vi "Google Earth.vi"() -> ()   [LabVIEW 2014]
uses:
  <vilib>/Instr/_visa.llb/VISA Configure Serial Port (Instr).vi
panel:
  out "Light":dbl(slide) scale=0.0..3000.0
  in  "Body Movements":T1
  out "Audio":dbl(slide) scale=0.0..30000.0
  out "x = y?":bool
  in  "Stop Button":bool
  in  "Globe Params":T2={"Longitude"=0.0, "Latitude"=0.0, "Altitude"=15000000.0, "Azimuth"=0.0}
  in  "Globe":refnum<k7>(container)
  in  "EARTHLib.IApplicationGE 2":refnum<k7>
  # "Space Glove Interface"
  # "Earth View"
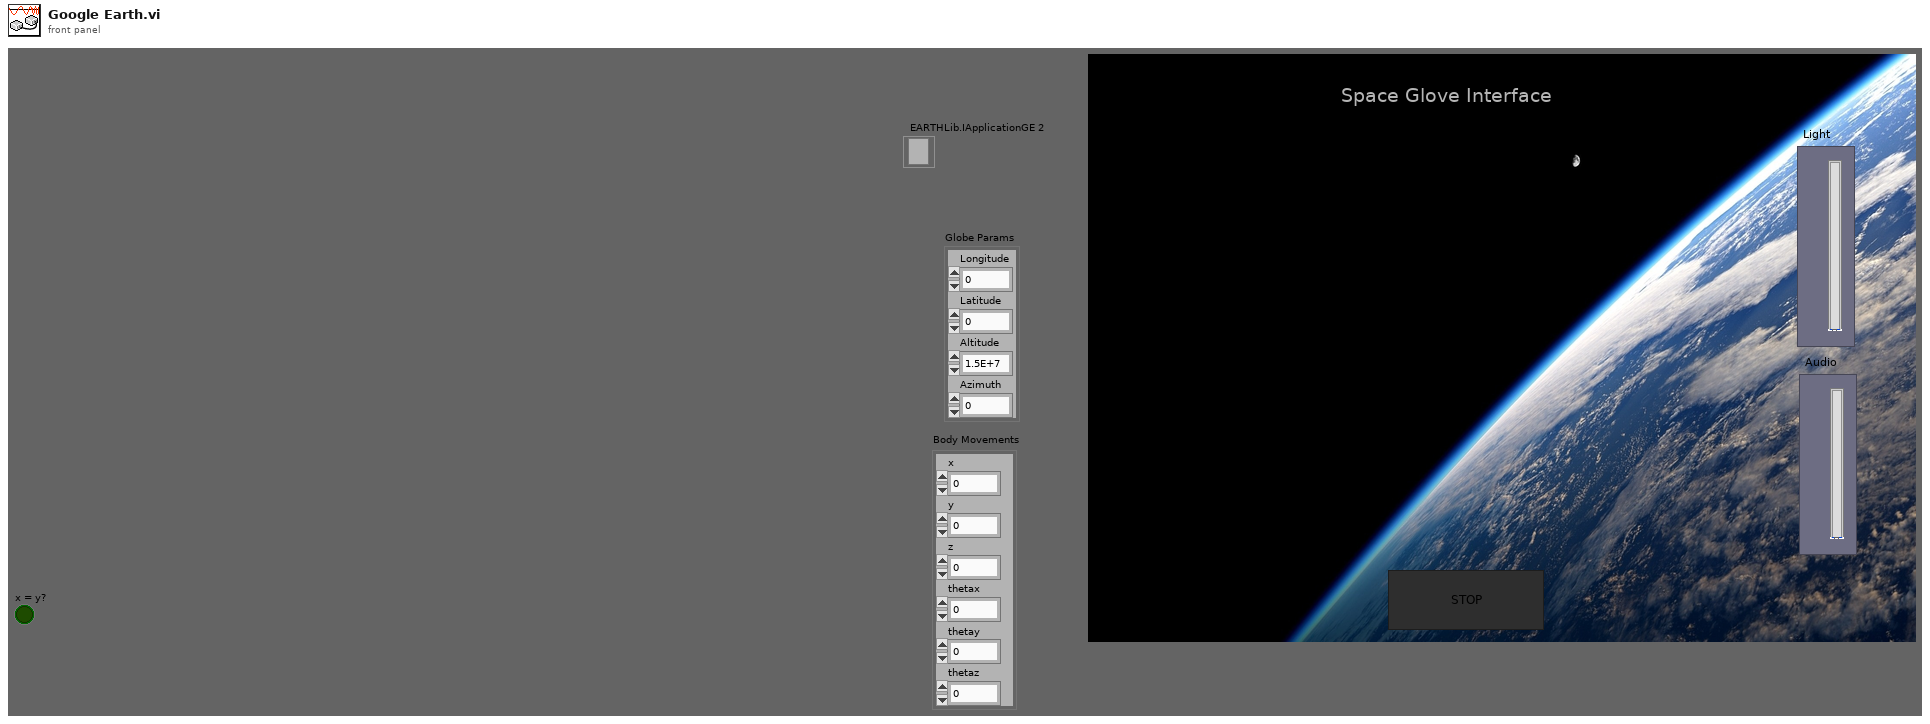
[diagram p1: front panel]
types:
  T1 = cluster{"x":sgl, "y":sgl, "z":sgl, "thetax":sgl, "thetay":sgl, "thetaz":sgl}
  T2 = cluster{"Longitude":dbl, "Latitude":dbl, "Altitude":dbl, "Azimuth":dbl}
  T3 = cluster{"Azimuth":dbl, "FocusPointAltitude":dbl, "altMode":i32, "FocusPointLatitude":dbl, "FocusPointLongitude":dbl, "Range":dbl, "Tilt":dbl}
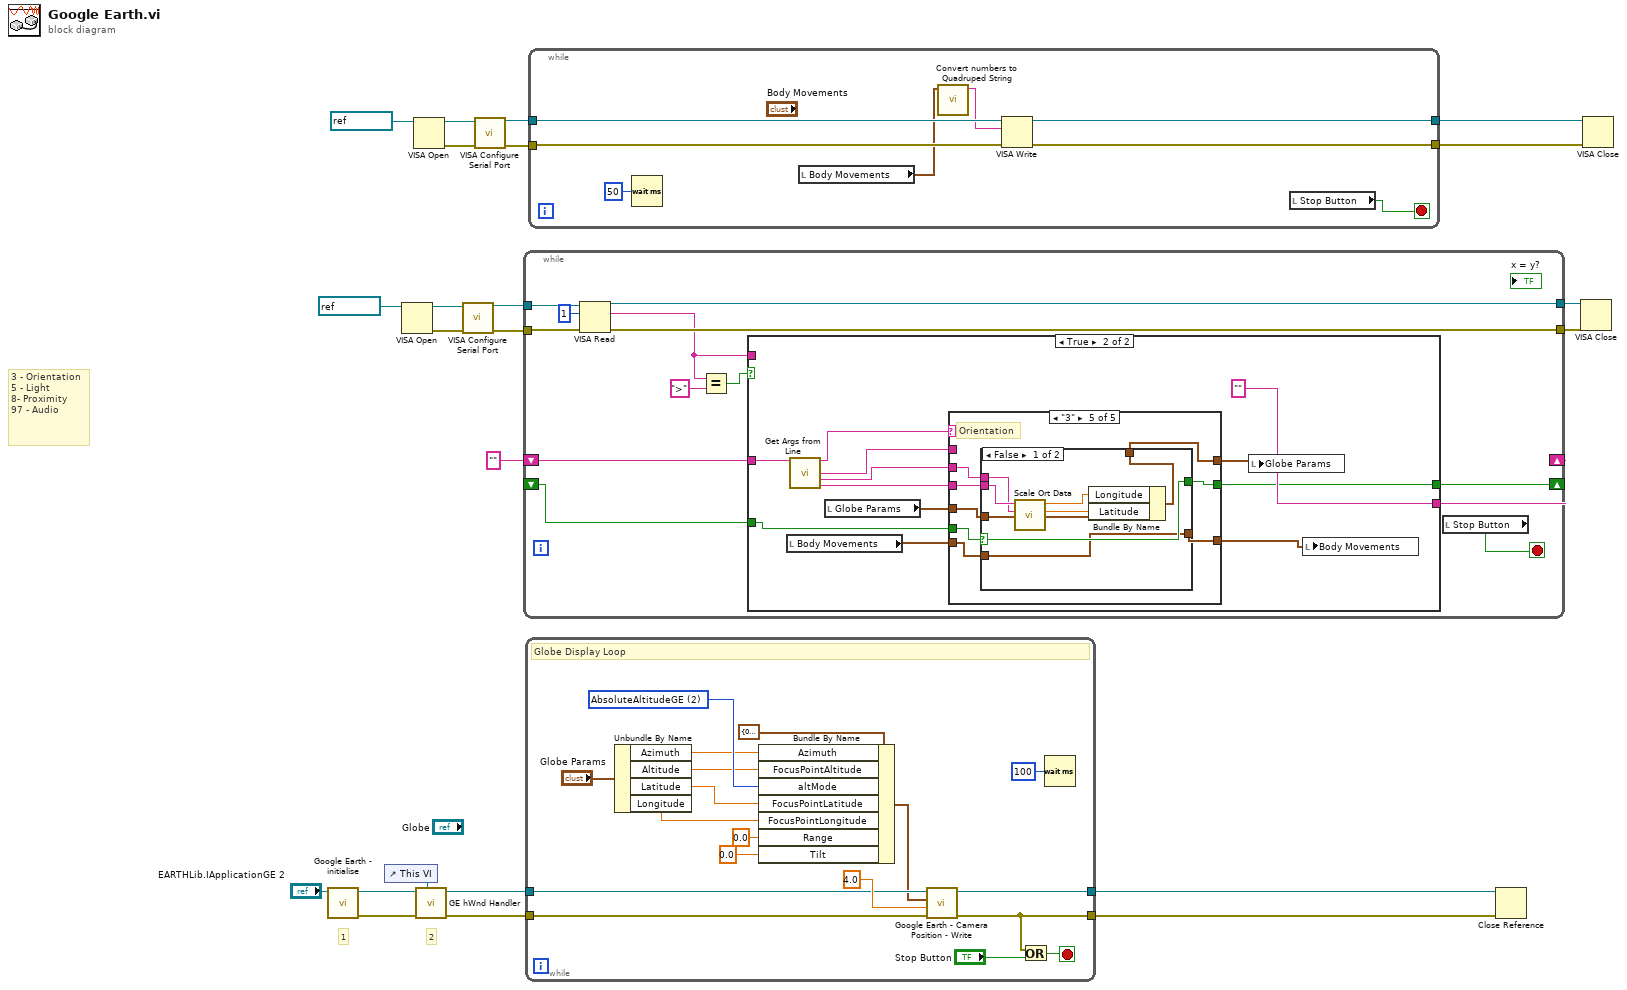
[diagram p0: block diagram]
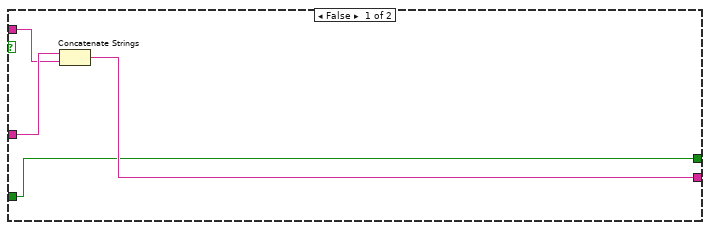
[diagram p2: hidden frame]
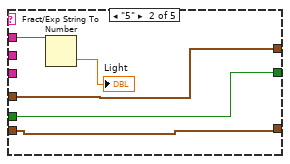
[diagram p4: hidden frame]
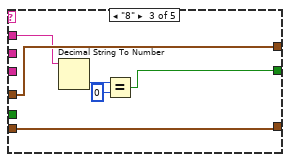
[diagram p5: hidden frame]
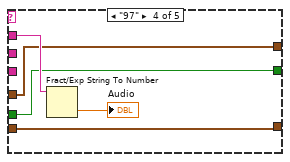
[diagram p6: hidden frame]
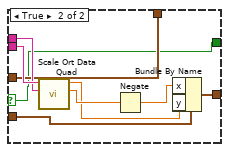
[diagram p7: hidden frame]
diagram:
  # "2"
  # "1"
  # "3 - Orientation\n5 - Light\n8- Proximity\n97 - Audio"
  n1 = call "Google Earth - initialise.vi"("EARTHLib.IApplicationGE"="EARTHLib.IApplicationGE 2") -> ("error out"=w22:errorcluster, "Refnum Out"=w21:refnum<k7>)  [unwired: 8 in, 1 out]
  n2 = control-ref of="This VI"() -> (w17:refnum<vi>)
  n3 = VISA Open(VISA resource name=refnum<visa-resource-name> "COM5") -> (VISA resource name=w14:refnum<visa-resource-name>, error out=w15:errorcluster)  [unwired: 4 in]
  n4 = VISA Open(VISA resource name=refnum<visa-resource-name> "COM4") -> (VISA resource name=w6:refnum<visa-resource-name>, error out=w7:errorcluster)  [unwired: 4 in]
  n5 = call "GE hWnd Handler.vi"("This VI"=w17, "error in"=w22, "Refnum In"=w21) -> ("error out"=w16:errorcluster, "Refnum Out"=w18:refnum<k7>)  [unwired: 7 in]
  n6 = call-poly "VISA Configure Serial Port"("VISA resource name"=w14, "error in (no error)"=w15) -> ("VISA resource name out"=w12:refnum<visa-resource-name>, "error out"=w11:errorcluster)  [unwired: 12 in]
  n7 = call-poly "VISA Configure Serial Port"("VISA resource name"=w6, "error in (no error)"=w7) -> ("VISA resource name out"=w4:refnum<visa-resource-name>, "error out"=w3:errorcluster)  [unwired: 12 in]
  n8 = while {
    tunnel: w12 -> [w36]
    tunnel: w11 -> [w35]
    tunnel: [w33] -> w10
    tunnel: [w32] -> w9
    shift-right: [w27] -> _
    shift-left: "" -> [w29]
    shift-right: [w25] -> _
    shift-left: _ -> [w24]
    stop <- w26 stop-if-true
    n9 = VISA Read(VISA resource name=w36, byte count=u32 1, error in (no error)=w35) -> (VISA resource name out=w32:refnum<visa-resource-name>, read buffer=w28:string, error out=w33:errorcluster)  [unwired: 1 out]
    n10 = Equal?(x=w28, y=">") -> (x = y?=w30:bool)
    n11 = case shown="True" w30 {
      tunnel: w29 -> [w39 w51]
      tunnel: w28 -> [w38 _]
      tunnel: [w40 ""] -> w27
      tunnel: [w37 w42] -> w25
      tunnel: w24 -> [w37 w41]
      frame False {
        n12 = Concatenate Strings(w39, w38) -> (w40:string)
      }
      frame True {
        n13 = local read "Body Movements"() -> (w44:T1)
        n14 = call "Get Args from Line.vi"("Data Line"=w51) -> ("Channel"=w50:string, "Arg1"=w48:string, "Arg2"=w47:string, "Arg3"=w46:string)  [unwired: 10 in, 1 out]
        n15 = local read "Globe Params"() -> (w49:T2)
        n16 = case shown="\"3\"" w50 {
          tunnel: w49 -> [w55 w57 w66 w70 w74]
          tunnel: w48 -> [_ w59 w64 w71 _]
          tunnel: w47 -> [_ _ _ _ w78]
          tunnel: w46 -> [_ _ _ _ w79]
          tunnel: [w55 w57 w66 w70 w73] -> w45
          tunnel: w44 -> [w54 w60 w65 w68 w77]
          tunnel: [w54 w60 w65 w68 w76] -> w43
          tunnel: [w53 w56 w61 w67 w72] -> w42
          tunnel: w41 -> [w53 w56 _ w67 w75]
          frame "False", Default {
          }
          frame "5" {
            n17 = Fract/Exp String To Number(string=w59) -> (number=→"Light":dbl)  [unwired: 3 in, 1 out]
          }
          frame "8" {
            n18 = Decimal String To Number(string=w64) -> (number=w63:i32)  [unwired: 2 in, 1 out]
            n19 = Equal?(x=w63, y=0) -> (x = y?=w61:bool)
          }
          frame "97" {
            n20 = Fract/Exp String To Number(string=w71) -> (number=→"Audio":dbl)  [unwired: 3 in, 1 out]
          }
          frame "3" {
            # "Orientation"
            n21 = case shown="False" w75 {
              selector: w75 -> [w81 w88]
              tunnel: w79 -> [w85 w96]
              tunnel: w78 -> [w84 w95]
              tunnel: w77 -> [w80 w94]
              tunnel: [w80 w92] -> w76
              tunnel: [w82 w89] -> w73
              tunnel: w74 -> [w83 w89]
              tunnel: [w81 w88] -> w72
              frame False {
                n22 = call "Scale Ort Data.vi"("Pitch (Arg 2)"=w84, "Roll (Arg 3)"=w85) -> ("Latitude"=w86:dbl, "Longitude"=w87:dbl)  [unwired: 8 in]
                n23 = Bundle By Name(cluster=w83, "Longitude"=w87, "Latitude"=w86) -> (w82:T2)
              }
              frame True {
                n24 = call "Scale Ort Data Quad.vi"("Pitch (Arg 2)"=w95, "Roll (Arg 3)"=w96) -> ("theta_y"=w93:dbl, "theta_x"=w90:dbl)  [unwired: 8 in]
                n25 = Negate(x=w93) -> (-x=w91:dbl)
                n26 = Bundle By Name(cluster=w94, "x"=w91, "y"=w90) -> (w92:T1)
              }
            }
          }
        }
        n27 = local write "Globe Params"(w45) -> ()
        n28 = local write "Body Movements"(w43) -> ()
      }
    }
    n29 = local read "Stop Button"() -> (w26:bool)
  }
  n30 = while {
    tunnel: w18 -> [w113]
    tunnel: [w111] -> w19
    tunnel: [w110] -> w20
    tunnel: w16 -> [w103]
    stop <- w112 stop-if-true
    w107 = 2 items=["RelativeToGroundAltitudeGE"=1, "AbsoluteAltitudeGE"=2] ("altMode")
    # "Globe Display Loop"
    n31 = Unbundle By Name("Globe Params") -> ("Azimuth"=w102:dbl, "Altitude"=w97:dbl, "Latitude"=w101:dbl, "Longitude"=w100:dbl)
    n32 = Bundle By Name(cluster=T3 {"Azimuth"=0.0, "FocusPointAltitude"=20000000.0, "altMode"=1, "FocusPointLatitude"=0.0, "FocusPointLongitude"=0.0, "Range"=0.0, "Tilt"=0.0} ("Camera Position"), "Azimuth"=w102, "FocusPointAltitude"=w97, "altMode"=w107, "FocusPointLatitude"=w101, "FocusPointLongitude"=w100, "Range"=0.0, "Tilt"=0.0) -> (w104:T3)
    n33 = call "Google Earth - Camera Position - Write.vi"("error in"=w103, "speed"=4.0 ("AutoPilotSpeed"), "Camera Position"=w104, "Refnum in"=w113) -> ("error out"=w111:errorcluster, "Refnum Out"=w110:refnum<k7>)  [unwired: 6 in]
    n34 = Or(x=w111, y="Stop Button") -> (x .or. y?=w112:bool)
    n35 = Wait (ms)(milliseconds to wait=u32 100) -> ()  [unwired: 1 out]
  }
  n36 = while {
    tunnel: w4 -> [w121]
    tunnel: w3 -> [w122]
    tunnel: [w118] -> w2
    tunnel: [w117] -> w1
    stop <- w120 stop-if-true
    n37 = Wait (ms)(milliseconds to wait=u32 50) -> ()  [unwired: 1 out]
    n38 = local read "Body Movements"() -> (w115:T1)
    n39 = call "Convert numbers to Quadruped String.vi"("Body Movements"=w115) -> ("String to Write to Quadruped"=w119:string)  [unwired: 10 in]
    n40 = VISA Write(VISA resource name=w121, write buffer=w119, error in (no error)=w122) -> (VISA resource name out=w118:refnum<visa-resource-name>, error out=w117:errorcluster)  [unwired: 1 out]
    n41 = local read "Stop Button"() -> (w120:bool)
  }
  n42 = Close Reference(reference=w20, error in (no error)=w19) -> ()  [unwired: 1 out]
  n43 = VISA Close(VISA resource name=w9, error in (no error)=w10) -> ()  [unwired: 1 out]
  n44 = VISA Close(VISA resource name=w2, error in (no error)=w1) -> ()  [unwired: 1 out]
